vi "Read ItemNames.vi"(8 "error in (no error)":errorcluster, 11 "BetterMultiListboxHandle in":refnum<class "BetterMultiListboxHandle.lvclass">) -> (0 "error out":errorcluster, 1 "Number of ItemNames":i32, 2 "Item Names":string[][](array[string]), 3 "BetterMultiListboxHandle out":refnum<class "BetterMultiListboxHandle.lvclass">)   [LabVIEW 2020, in "BetterDragAndDrop.lvlib" / "BetterMultiListboxHandle.lvclass"]
uses:
  BetterMultiListboxHandle.lvclass
  BetterMultiListboxHandle.lvclass/BetterMultiListboxHandle.ctl
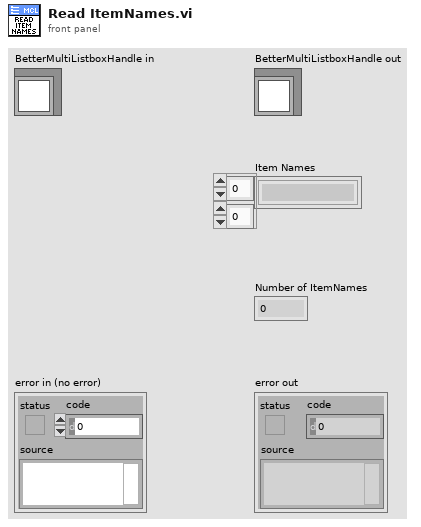
[diagram p1: front panel]
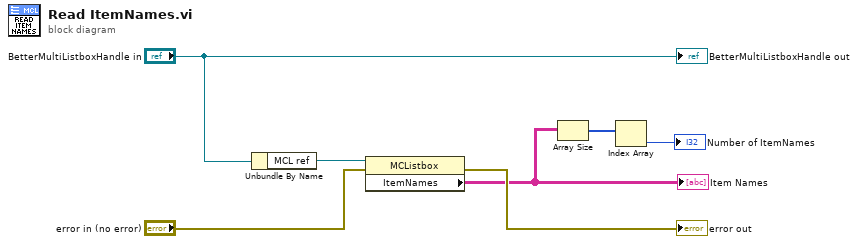
[diagram p0: block diagram]
diagram:
  n1 = Unbundle By Name("BetterMultiListboxHandle in") -> ("MCL ref"=w6:refnum<vi>)
  n2 = property class="MCListbox"(reference=w6, error in="error in (no error)") -> (error out=→"error out":errorcluster, "ItemNames"=w2:string[][])  [unwired: 1 out]
  "Item Names" <- w2
  n3 = Array Size(array=w2) -> (size(s)=w3:i32[])
  n4 = Index Array(array=w3) -> (element=→"Number of ItemNames":i32)  [unwired: 1 in]
  "BetterMultiListboxHandle out" <- "BetterMultiListboxHandle in"
